vi "Reinit diagnostics references.vi"(8 "error in (no error)":errorcluster, 11 "ZenGage v3.0 UI in":T1) -> (0 "error out":errorcluster)   [LabVIEW 2019, in "ZenGage v3.0 UI.lvclass"]
uses:
  ZenGage v3.0 UI.lvclass
  Type Definitions/Controls and Indicators/Select a part (combobox).ctl
  Type Definitions/Controls and Indicators/EDL control references.ctl
  Type Definitions/Controls and Indicators/Diagnostics control referencs.ctl
  Type Definitions/Controls and Indicators/Inspection control references.ctl
  Type Definitions/Controls and Indicators/General_Control references.ctl
  Type Definitions/Controls and Indicators/Controls and Indicators Cluster.ctl
  Type Definitions/General/Master sample references.ctl
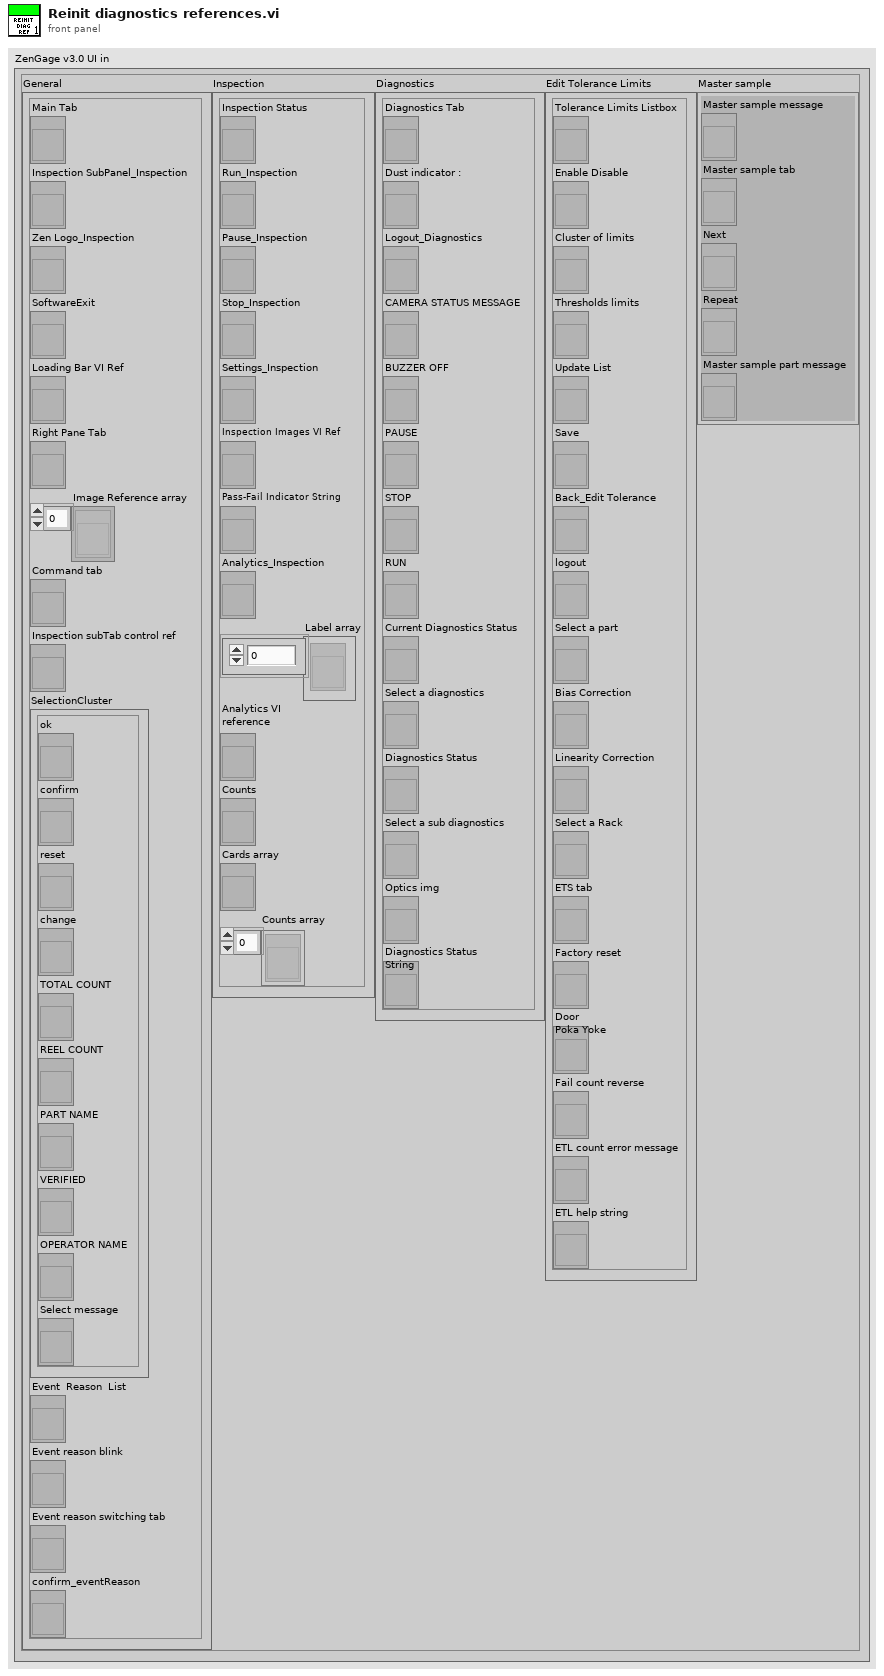
[diagram p1: front panel]
types:
  T1 = typedef "ZenGage v3.0 UI.lvclass/Controls and Indicators Cluster.ctl" = cluster{"General":T2, "Inspection":T3, "Diagnostics":T4, "Edit Tolerance Limits":T5, "Master sample":T6}
  T2 = typedef "ZenGage v3.0 UI.lvclass/General_Control references.ctl" = cluster{"Main Tab":refnum<vi>, "Inspection SubPanel_Inspection":refnum<vi>, "Zen Logo_Inspection":refnum<vi>, "SoftwareExit":refnum<vi>, "Loading Bar VI Ref":refnum<vi>, "Right Pane Tab":refnum<vi>, "Image Reference array":refnum<vi>[], "Command tab":refnum<vi>, "Inspection subTab control ref":refnum<vi>, "SelectionCluster":cluster{"ok":refnum<vi>, "confirm":refnum<vi>, "reset":refnum<vi>, "change":refnum<vi>, "TOTAL COUNT":refnum<vi>, "REEL COUNT":refnum<vi>, "PART NAME":refnum<vi>, "VERIFIED":refnum<vi>, "OPERATOR NAME":refnum<vi>, "Select message":refnum<vi>}, "Event  Reason  List":refnum<vi>, "Event reason blink":refnum<vi>, "Event reason switching tab":refnum<vi>, "confirm_eventReason":refnum<vi>}
  T3 = typedef "ZenGage v3.0 UI.lvclass/Inspection control references.ctl" = cluster{"Inspection Status":refnum<vi>, "Run_Inspection":refnum<vi>, "Pause_Inspection":refnum<vi>, "Stop_Inspection":refnum<vi>, "Settings_Inspection":refnum<vi>, "Inspection Images VI Ref":refnum<vi>, "Pass-Fail Indicator String":refnum<vi>, "Analytics_Inspection":refnum<vi>, "Label array":refnum<vi>[], "Analytics VI\nreference":refnum<vi>, "Counts":refnum<vi>, "Cards array":refnum<vi>, "Counts array":refnum<vi>[]}
  T4 = typedef "ZenGage v3.0 UI.lvclass/Diagnostics control referencs.ctl" = cluster{"Diagnostics Tab":refnum<vi>, "Dust indicator :":refnum<vi>, "Logout_Diagnostics":refnum<vi>, "CAMERA STATUS MESSAGE":refnum<vi>, "BUZZER OFF":refnum<vi>, "PAUSE":refnum<vi>, "STOP":refnum<vi>, "RUN":refnum<vi>, "Current Diagnostics Status":refnum<vi>, "Select a diagnostics":refnum<vi>, "Diagnostics Status":refnum<vi>, "Select a sub diagnostics":refnum<vi>, "Optics img":refnum<vi>, "Diagnostics Status\nString":refnum<vi>}
  T5 = typedef "ZenGage v3.0 UI.lvclass/EDL control references.ctl" = cluster{"Tolerance Limits Listbox":refnum<vi>, "Enable Disable":refnum<vi>, "Cluster of limits":refnum<vi>, "Thresholds limits":refnum<vi>, "Update List":refnum<vi>, "Save":refnum<vi>, "Back_Edit Tolerance":refnum<vi>, "logout":refnum<vi>, "Select a part":refnum<vi>, "Bias Correction":refnum<vi>, "Linearity Correction":refnum<vi>, "Select a Rack":refnum<vi>, "ETS tab":refnum<vi>, "Factory reset":refnum<vi>, "Door\nPoka Yoke":refnum<vi>, "Fail count reverse":refnum<vi>, "ETL count error message":refnum<vi>, "ETL help string":refnum<vi>}
  T6 = typedef "Master sample references.ctl" = cluster{"Master sample message":refnum<vi>, "Master sample tab":refnum<vi>, "Next":refnum<vi>, "Repeat":refnum<vi>, "Master sample part message":refnum<vi>}
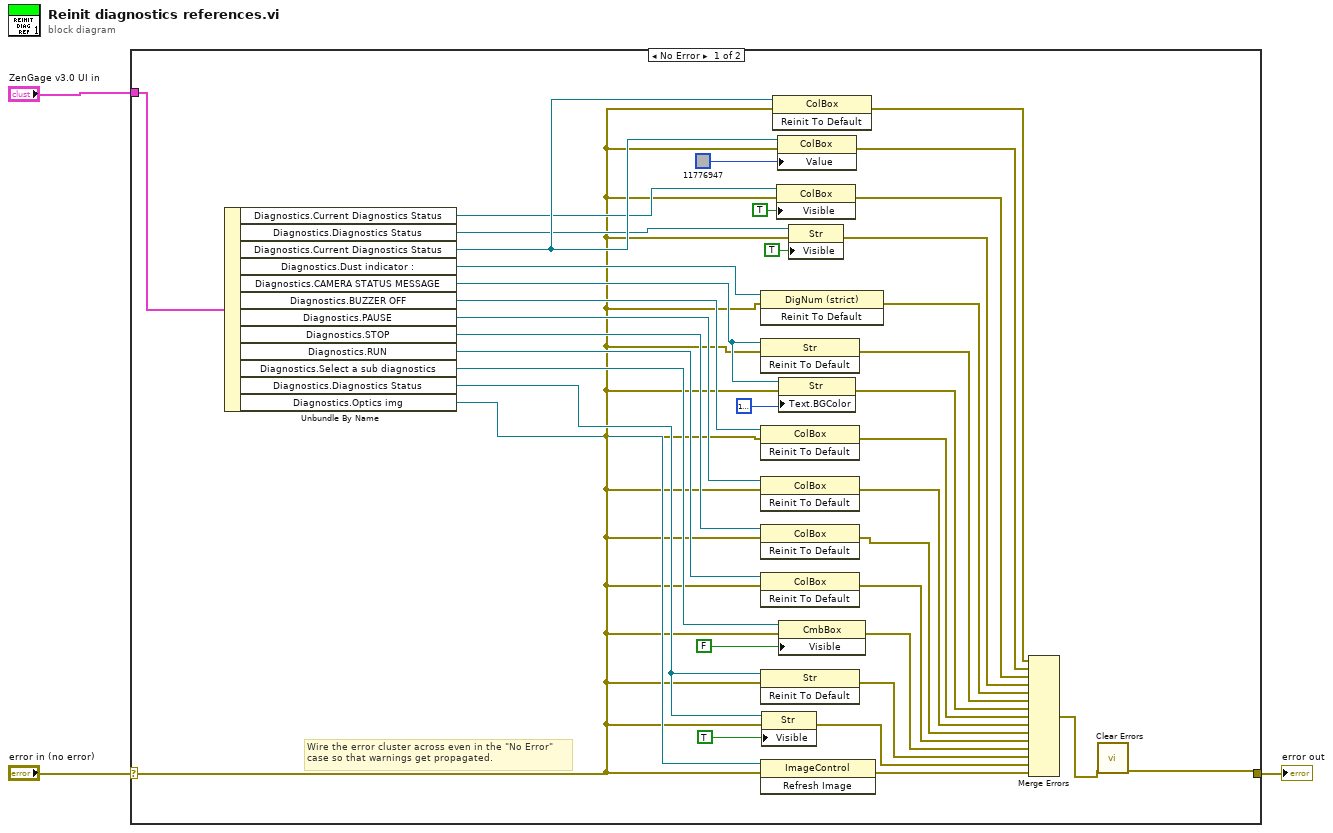
[diagram p0: block diagram]
diagram:
  n1 = case shown="No Error" "error in (no error)" {
    selector: "error in (no error)" -> [w6 w41]
    tunnel: [w24 w41] -> w2
    tunnel: "ZenGage v3.0 UI in" -> [w40 _]
    frame No Error {
      # "Wire the error cluster across even in the \"No Error\"\ncase so that warnings get propagated."
      n2 = Unbundle By Name(w40) -> ("Diagnostics.Current Diagnostics Status"=w9:refnum<vi>, "Diagnostics.Diagnostics Status"=w10:refnum<vi>, "Diagnostics.Current Diagnostics Status"=w11:refnum<vi>, "Diagnostics.Dust indicator :"=w39:refnum<vi>, "Diagnostics.CAMERA STATUS MESSAGE"=w18:refnum<vi>, "Diagnostics.BUZZER OFF"=w38:refnum<vi>, "Diagnostics.PAUSE"=w37:refnum<vi>, "Diagnostics.STOP"=w36:refnum<vi>, "Diagnostics.RUN"=w35:refnum<vi>, "Diagnostics.Select a sub diagnostics"=w34:refnum<vi>, "Diagnostics.Diagnostics Status"=w23:refnum<vi>, "Diagnostics.Optics img"=w33:refnum<vi>)
      n3 = invoke class="DigNum (strict)" method="Reinit To Default"(reference=w39, error in=w6) -> (error out=w15:errorcluster)  [unwired: 1 in, 2 out]
      n4 = invoke class="Str" method="Reinit To Default"(reference=w18, error in=w6) -> (error out=w14:errorcluster)  [unwired: 1 in, 2 out]
      n5 = invoke class="ColBox" method="Reinit To Default"(reference=w38, error in=w6) -> (error out=w13:errorcluster)  [unwired: 1 in, 2 out]
      n6 = invoke class="ColBox" method="Reinit To Default"(reference=w37, error in=w6) -> (error out=w26:errorcluster)  [unwired: 1 in, 2 out]
      n7 = invoke class="ColBox" method="Reinit To Default"(reference=w36, error in=w6) -> (error out=w27:errorcluster)  [unwired: 1 in, 2 out]
      n8 = invoke class="ColBox" method="Reinit To Default"(reference=w35, error in=w6) -> (error out=w28:errorcluster)  [unwired: 1 in, 2 out]
      n9 = invoke class="Str" method="Reinit To Default"(reference=w23, error in=w6) -> (error out=w30:errorcluster)  [unwired: 1 in, 2 out]
      n10 = invoke class="ImageControl" method="Refresh Image"(reference=w33, error in=w6) -> (error out=w31:errorcluster)  [unwired: 1 in, 2 out]
      n11 = property class="Str"(reference=w23, error in=w6, "Visible"=TRUE) -> (error out=w21:errorcluster)  [unwired: 1 out]
      n12 = invoke class="ColBox" method="Reinit To Default"(reference=w11, error in=w6) -> (error out=w20:errorcluster)  [unwired: 1 in, 2 out]
      n13 = property class="ColBox"(reference=w9, error in=w6, "Visible"=TRUE) -> (error out=w5:errorcluster)  [unwired: 1 out]
      n14 = property class="ColBox"(reference=w11, error in=w6, "Value"=u32 11776947) -> (error out=w16:errorcluster)  [unwired: 1 out]
      n15 = property class="Str"(reference=w18, error in=w6, "Text.BGColor"=u32 16777216) -> (error out=w12:errorcluster)  [unwired: 1 out]
      n16 = property class="CmbBox"(reference=w34, error in=w6, "Visible"=FALSE) -> (error out=w29:errorcluster)  [unwired: 1 out]
      n17 = property class="Str"(reference=w10, error in=w6, "Visible"=TRUE) -> (error out=w4:errorcluster)  [unwired: 1 out]
      n18 = Merge Errors(w20, w16, w5, w4, w15, w14, w12, w13, w26, w27, w28, w29, w30, w21, w31) -> (w25:errorcluster)
      n19 = call <vilib>:"Clear Errors.vi"("error in (no error)"=w25) -> ("error out"=w24:errorcluster)  [unwired: 5 in, 1 out]
    }
    frame Error {
    }
  }
  "error out" <- w2
